vi "Verify Scripting Code.vi"(8 "error in":errorcluster) -> (0 "error out":errorcluster)   [LabVIEW 2020, in "Caraya Extension Tests.lvclass"]
uses:
  Caraya Extension Tests.lvclass
  <vilib>/addons/_JKI Toolkits/Caraya/classes/Test/Test.lvclass
  Source/Extensions/Caraya.Extension/Caraya.Extension.lvlib
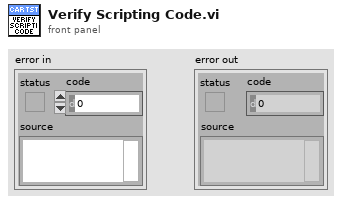
[diagram p1: front panel]
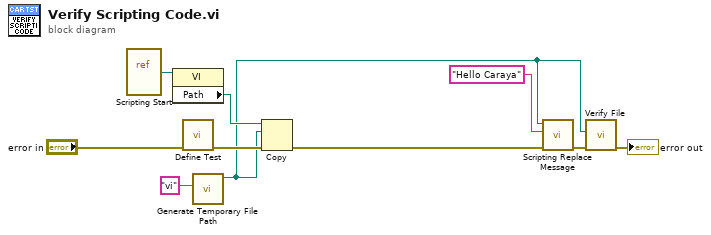
[diagram p0: block diagram]
diagram:
  n1 = vi-ref "Scripting Start.vi"() -> (w5:refnum<vi>)
  n2 = property on="Property Node" class="VI"(reference=w5) -> ("Path"=w2:path)  [unwired: 1 in, 2 out]
  n3 = call <vilib>:"Define Test.vi"("error in (no error)"="error in") -> ("error out"=w7:errorcluster)  [unwired: 9 in, 1 out]
  n4 = call <vilib>:"Generate Temporary File Path.vi"("Temporary File Extension (tmp)"="vi") -> ("Unique Temporary File Path"=w1:path)  [unwired: 9 in, 1 out]
  n5 = Copy(8:w7, 10:w1, 11:w2) -> (0:w6:errorcluster)  [unwired: 2 in, 2 out]
  n6 = call "Scripting Replace Message.vi"("error in"=w6, "New Message"="Hello Caraya", "Path"=w1) -> ("error out"=w8:errorcluster)  [unwired: 8 in]
  n7 = call "Verify File.vi"("error in"=w8, "path to file"=w1) -> ("error out"=→"error out":errorcluster)  [unwired: 8 in, 1 out]
